vi "Validate Dynamic Config.vi"(10 "SignalIDs":i32[](array[numeric]), 11 "Response Ref in":refnum<queue>) -> (2 "Response Ref out":refnum<queue>, 3 "Dynamic Config Status":bool)   [LabVIEW 2025, in "Runtime Configuration Support Example Engine.lvlib"]
uses:
  Runtime Configuration Support Example Engine.lvlib
  HW Operations.ctl
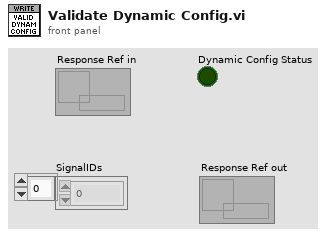
[diagram p1: front panel]
types:
  T1 = typedef "HW Operations.ctl" = enum16{"Initialize", "Set In Val", "Get In Val", "Set Block", "Set Out Val", "Get Out Val", "Get In Array", "Get Out Array"}
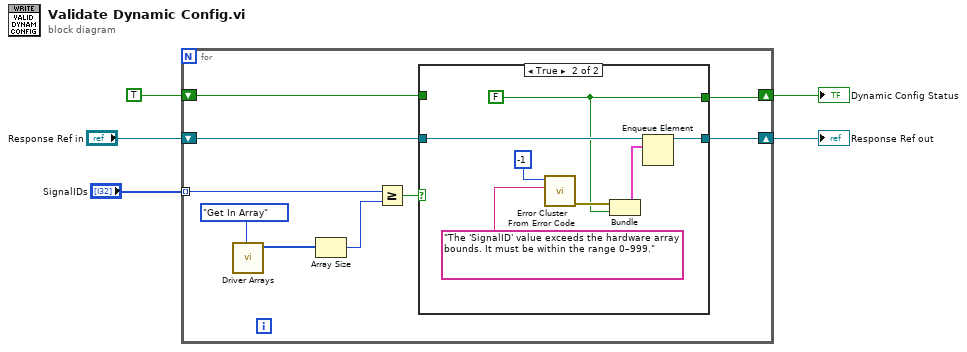
[diagram p0: block diagram]
diagram:
  n1 = for {
    tunnel: "SignalIDs" -> [w14] mode=indexing
    shift-right: [w11] -> w3
    shift-left: "Response Ref in" -> [w12]
    shift-right: [w9] -> w1
    shift-left: TRUE -> [w10]
    n2 = call "Driver Arrays.vi"("Curr Operation"=HW_Operations."Get In Array") -> ("Inport arr"=w7:i32[])  [unwired: 7 in, 3 out]
    n3 = Array Size(array=w7) -> (size(s)=w8:i32)
    n4 = Greater Or Equal?(x=w14, y=w8) -> (x >= y?=w13:bool)
    n5 = case shown="True" w13 {
      tunnel: w12 -> [w16 w20]
      tunnel: [w16 w18] -> w11
      tunnel: w10 -> [w15 _]
      tunnel: [w15 w17] -> w9
      frame False {
      }
      frame True {
        w17 = FALSE
        n6 = call <vilib>:"Error Cluster From Error Code.vi"("error message (\"\")"="The 'SignalID' value exceeds the hardware array bounds. It must be within the range 0–999." ("error message (\"\")"), "error code (0)"=-1) -> ("error out"=w23:errorcluster)  [unwired: 7 in]
        n7 = Bundle("error out"=w23, w17) -> (w19:cluster{"error out":errorcluster, bool})  [unwired: 1 in]
        n8 = Enqueue Element(queue=w20, element=w19) -> (queue out=w18:refnum<queue>)  [unwired: 2 in, 2 out]
      }
    }
  }
  "Response Ref out" <- w3
  "Dynamic Config Status" <- w1
